vi "decimate.vi"(9 "offset":u16, 10 "decimation":u16, 11 "run flags":u8) -> (1 "new offset":u16, 2 "decimation out":u16, 3 "run flags out":u8)   [LabVIEW 2013, in "main engine.lvlib"]
uses:
  main engine.lvlib
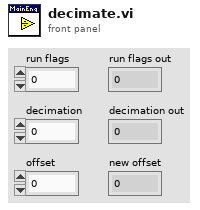
[diagram p1: front panel]
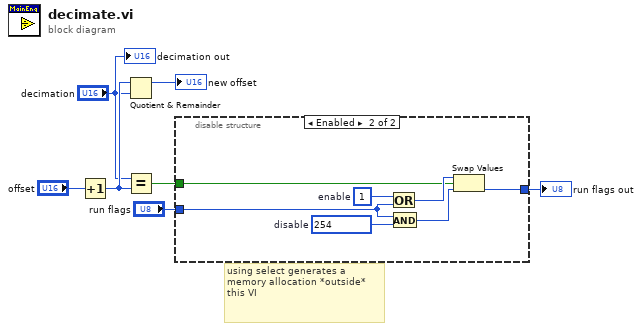
[diagram p0: block diagram]
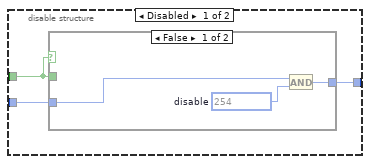
[diagram p2: hidden frame]
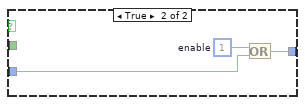
[diagram p3: hidden frame]
diagram:
  # "using select generates a memory allocation *outside* this VI"
  n1 = Increment(x="offset") -> (x+1=w6:u16)
  n2 = Quotient & Remainder(x=w6, y="decimation") -> (x-y*floor(x/y)=→"new offset":u16)  [unwired: 1 out]
  n3 = Equal?(x="decimation", y=w6) -> (x = y?=w1:bool)
  n4 = disable-structure shown="Enabled" {
    disable-tunnel: "run flags" -> [w10 w19]
    disable-tunnel: [w9 w17] -> w2
    disable-tunnel: w1 -> [w8 w18]
    frame Disabled {
      n5 = case shown="False" w8 {
        tunnel: w8 -> [_ _]
        tunnel: w10 -> [w13 w16]
        tunnel: [w11 w14] -> w9
        frame False {
          w12 = u8 254  # disable
          n6 = And(x=w13, y=w12) -> (x .and. y?=w11:u8)
        }
        frame True {
          w15 = u8 1  # enable
          n7 = Or(x=w15, y=w16) -> (x .or. y?=w14:u8)
        }
      }
    }
    frame Enabled {
      w21 = u8 254  # disable
      w20 = u8 1  # enable
      n8 = Or(x=w20, y=w19) -> (x .or. y?=w22:u8)
      n9 = And(x=w19, y=w21) -> (x .and. y?=w23:u8)
      n10 = Swap Values(12:w22, 13:w18, 14:w23) -> (3:w17:u8)  [unwired: 1 out]
    }
  }
  "run flags out" <- w2
  "decimation out" <- "decimation"
